vi "_RT_CtrlLoop_D999_SystemInit.vi"(3 "VISA resource In":refnum<visa-resource-name>, 4 "Head+Addr+Seg":string, 5 "Init Value":T1={"Enable"=FALSE, "AI"=[{"Label"="", "MultiValue"=1.0, "AddValue"=0.0}, {"Label"="", "MultiValue"=1.0, "AddValue"=0.0}, {"Label"="", "MultiValue"=1.0, "AddValue"=0.0}, {"Label"="", "MultiValue"=1.0, "AddValue"=0.0}, {"Label"="", "MultiValue"=1.0, "AddValue"=0.0}, {"Label"="", "MultiValue"=1.0, "AddValue"=0.0}, {"Label"="", "MultiValue"=1.0, "AddValue"=0.0}, {"Label"="", "MultiValue"=1.0, "AddValue"=0.0}, {"Label"="", "MultiValue"=1.0, "AddValue"=0.0}, {"Label"="", "MultiValue"=1.0, "AddValue"=0.0}, {"Label"="", "MultiValue"=1.0, "AddValue"=0.0}, {"Label"="", "MultiValue"=1.0, "AddValue"=0.0}], "AO"=[], "Switch"=[]}) -> (0 "Finish?":bool, 2 "Return Value":T1={"Enable"=FALSE, "AI"=[{"Label"="", "MultiValue"=1.0, "AddValue"=0.0}, {"Label"="", "MultiValue"=1.0, "AddValue"=0.0}, {"Label"="", "MultiValue"=1.0, "AddValue"=0.0}, {"Label"="", "MultiValue"=1.0, "AddValue"=0.0}, {"Label"="", "MultiValue"=1.0, "AddValue"=0.0}, {"Label"="", "MultiValue"=1.0, "AddValue"=0.0}, {"Label"="", "MultiValue"=1.0, "AddValue"=0.0}, {"Label"="", "MultiValue"=1.0, "AddValue"=0.0}, {"Label"="", "MultiValue"=1.0, "AddValue"=0.0}, {"Label"="", "MultiValue"=1.0, "AddValue"=0.0}, {"Label"="", "MultiValue"=1.0, "AddValue"=0.0}, {"Label"="", "MultiValue"=1.0, "AddValue"=0.0}], "AO"=[], "Switch"=[]})   [LabVIEW 2018]
uses:
  PublicSubVI/Ctl/_ctl_RT_D999_Param.ctl
  PublicSubVI/Ctl/_ctl_RT_D999_Settings.ctl
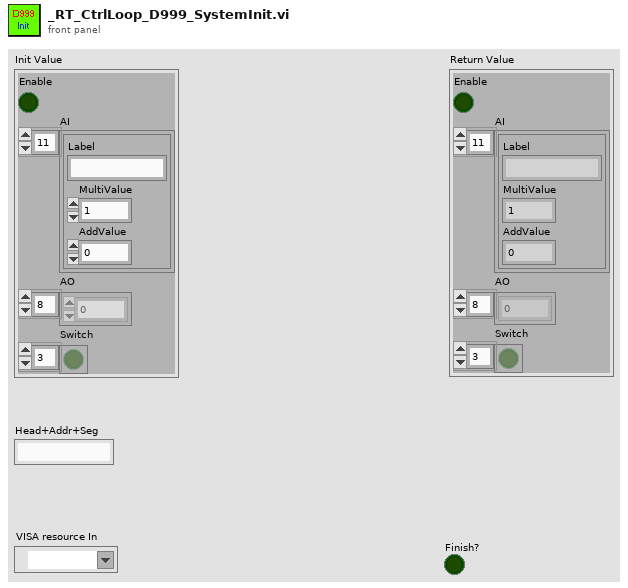
[diagram p1: front panel]
types:
  T1 = typedef "_ctl_RT_D999_Param.ctl" = cluster{"Enable":bool, "AI":cluster{"Label":string, "MultiValue":dbl, "AddValue":dbl}[], "AO":i16[], "Switch":bool[]}
  T2 = enum16{"None", "Init", "Write", "WriteAll", "Read", "ReadAll", "SetEnable", "SetParam", "ReadAO", "ReadSwitch"}
  T3 = typedef "_ctl_RT_D999_Settings.ctl" = cluster{"Cmd":enum16{"None", "Init", "Write", "WriteAll", "Read", "ReadAll", "SetEnable", "SetParam", "ReadAO", "ReadSwitch", "ReportID"}, "Variant":variant}
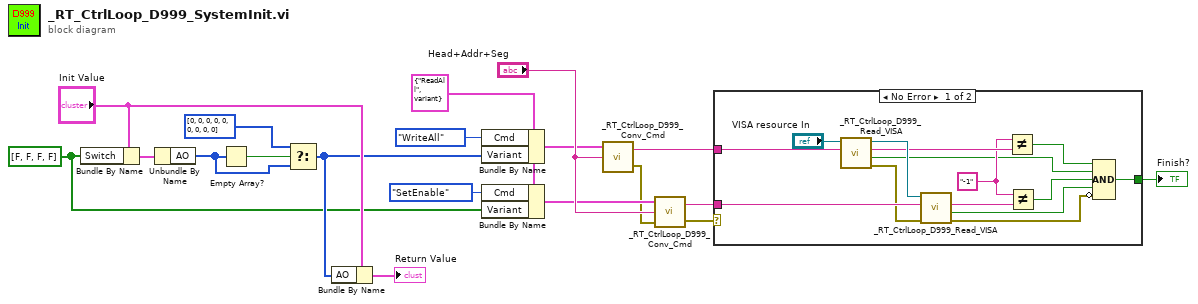
[diagram p0: block diagram]
diagram:
  w1 = bool[] [FALSE, FALSE, FALSE, FALSE] ("Switch")
  w9 = T3 {"Cmd"=enum."ReadAll", "Variant"=variant} ("CmdParam")
  n1 = Bundle By Name(cluster="Init Value", "Switch"=w1) -> (w14:T1)
  n2 = Unbundle By Name(w14) -> ("AO"=w16:i16[])
  n3 = Empty Array?(array=w16) -> (empty?=w17:bool)
  n4 = Select(t=i16[] [0, 0, 0, 0, 0, 0, 0, 0, 0], s=w17, f=w16) -> (s? t:f=w11:i16[])
  n5 = Bundle By Name(cluster="Init Value", "AO"=w11) -> (→"Return Value":T1)
  n6 = Bundle By Name(cluster=w9, "Cmd"=T2."WriteAll", "Variant"=w11) -> (w7:T3)
  n7 = Bundle By Name(cluster=w9, "Cmd"=T2."SetEnable", "Variant"=w1) -> (w6:T3)
  n8 = call "_RT_CtrlLoop_D999_Conv_Cmd.vi"("Head+Addr+Seg"="Head+Addr+Seg", "CmdParam"=w7) -> ("error out"=w5:errorcluster, "Cmd_String"=w2:string)  [unwired: 1 in]
  n9 = call "_RT_CtrlLoop_D999_Conv_Cmd.vi"("error in (no error)"=w5, "Head+Addr+Seg"="Head+Addr+Seg", "CmdParam"=w6) -> ("error out"=w4:errorcluster, "Cmd_String"=w3:string)
  n10 = case shown="No Error" w4 {
    tunnel: w2 -> [w32 _]
    tunnel: w3 -> [w31 _]
    tunnel: [w20 _] -> w19
    frame No Error {
      w26 = "-1"
      n11 = call "_RT_CtrlLoop_D999_Read_VISA.vi"("Comm Str"=w32, "VISA resource In"="VISA resource In") -> ("error out"=w29:errorcluster, "Is Exist?"=w24:bool, "Response Str"=w27:string, "VISA resource Out"=w30:refnum<visa-resource-name>)  [unwired: 6 in]
      n12 = call "_RT_CtrlLoop_D999_Read_VISA.vi"("error in (no error)"=w29, "Comm Str"=w31, "VISA resource In"=w30) -> ("error out"=w21:errorcluster, "Is Exist?"=w22:bool, "Response Str"=w28:string)  [unwired: 5 in, 1 out]
      n13 = Not Equal?(x=w26, y=w27) -> (x != y?=w25:bool)
      n14 = Not Equal?(x=w26, y=w28) -> (x != y?=w23:bool)
      n15 = Compound Arithmetic op=AND(w25, w24, w23, w22, invert w21) -> (w20:bool)
    }
    frame Error {
    }
  }
  "Finish?" <- w19
